vi "Test Sinewave Class.vi"(8 "error in":errorcluster, 11 "TestCase in":refnum<class "Test FGEN.lvclass">) -> (0 "error out":errorcluster, 3 "TestCase out":refnum<class "Test FGEN.lvclass">)   [LabVIEW 2020, in "Test FGEN.lvclass"]
uses:
  Test FGEN.lvclass
  Libraries/FGen/Clases/Generador/Generador.lvclass
  <vilib>/addons/_JKI Toolkits/VI Tester/TestCase.llb/TestCase.lvclass
  <vilib>/measure/NI_MABase.lvlib
  C:/Program Files (x86)/National Instruments/LabVIEW 2020/vi.lib/addons/_JKI Toolkits/VI Tester/TestCase.llb/TestCase.lvclass
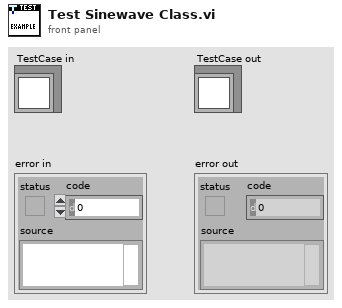
[diagram p1: front panel]
types:
  T1 = enum16{"Sine Wave", "Triangle Wave", "Square Wave", "Sawtooth Wave"}
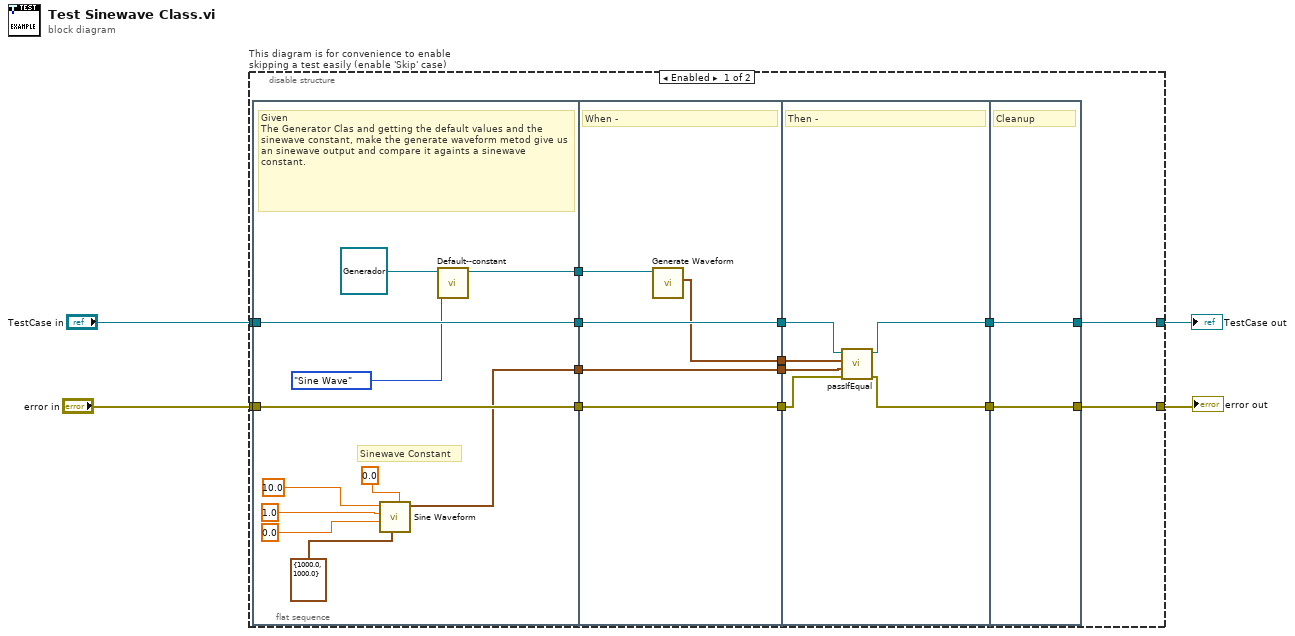
[diagram p0: block diagram]
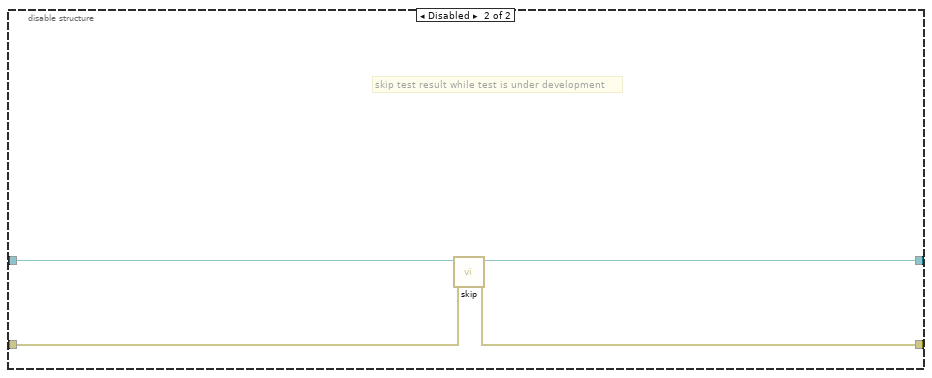
[diagram p2: hidden frame]
diagram:
  n1 = disable-structure "This diagram is for convenience to enable skipping a test easily (enable 'Skip' case)" shown="Enabled" {
    disable-tunnel: "TestCase in" -> [w10 w44]
    disable-tunnel: [w9 w43] -> w1
    disable-tunnel: [w17 w46] -> w3
    disable-tunnel: "error in" -> [w16 w45]
    frame Enabled {
      n2 = flat-sequence {
        tunnel: w10 -> [w28]
        tunnel: [w28] -> w13
        tunnel: w16 -> [w29]
        tunnel: [w29] -> w14
        tunnel: [w26] -> w8
        tunnel: [w20] -> w5
        tunnel: [w33] -> w12
        tunnel: w13 -> [w33]
        tunnel: [w34] -> w15
        tunnel: w14 -> [w34]
        tunnel: w8 -> [w32]
        tunnel: [w31] -> w7
        tunnel: [w30] -> w6
        tunnel: w5 -> [w30]
        tunnel: [w37] -> w11
        tunnel: [w40] -> w18
        tunnel: w12 -> [w38]
        tunnel: w15 -> [w39]
        tunnel: w7 -> [w36]
        tunnel: w6 -> [w35]
        tunnel: [w42] -> w17
        tunnel: [w41] -> w9
        tunnel: w11 -> [w41]
        tunnel: w18 -> [w42]
        frame #0 {
          # "Sinewave Constant"
          # "Given\nThe Generator Clas and getting the default values and the sinewave constant, make the generate waveform metod give us an sinewave output and compare it againts a sinewave constant."
          n3 = call <vilib>:"Sine Waveform.vi"("offset"=0.0, "sampling info"=cluster{"Fs":dbl, "#s":dbl} {"Fs"=1000.0, "#s"=1000.0}, "phase"=0.0, "amplitude"=1.0, "frequency"=10.0) -> ("signal out"=w20:waveform(dbl))  [unwired: 5 in, 1 out]
          n4 = call-dynamic "Default--constant.vi"("signal type"=T1."Sine Wave", "Generator in"=refnum<class "Generador.lvclass"> refnum ("FGen.lvlib:Generator")) -> ("Generator out"=w26:refnum<class "Generador.lvclass">)  [unwired: 8 in, 1 out]
        }
        frame #1 {
          # "When -"
          n5 = call "Generate Waveform.vi"("Generator in"=w32) -> ("Waveform"=w31:waveform(dbl))  [unwired: 8 in, 2 out]
        }
        frame #2 {
          # "Then -"
          n6 = call-dynamic "passIfEqual.vi"("error in (no error)"=w39, "y"=w35, "x"=w36, "TestCase in"=w38) -> ("error out"=w40:errorcluster, "TestCase out"=w37:refnum<class "Test FGEN.lvclass">)  [unwired: 6 in]
        }
        frame #3 {
          # "Cleanup"
        }
      }
    }
    frame Disabled {
      # "skip test result while test is under development"
      n7 = call <vilib>:"skip.vi"("error in (no error)"=w45, "TestCase in"=w44) -> ("error out"=w46:errorcluster, "TestCase out"=w43:refnum<class "Test FGEN.lvclass">)  [unwired: 8 in]
    }
  }
  "error out" <- w3
  "TestCase out" <- w1
